vi "Open Connection (ODBC).vi"(8 "error in (no error)":errorcluster, 9 "password":string, 10 "userID":string, 11 "DSN Name":string) -> (0 "error out":errorcluster, 3 "connection reference":T1)   [LabVIEW 2020, in "Oracle Driver.lvlib"]
uses:
  Oracle Driver.lvlib
  <vilib>/addons/database/Connection.llb/Conn ObjectReference.ctl
  <vilib>/addons/database/Connection.llb/DB Tools Open Connec (String).vi
  <vilib>/addons/database/NI_Database_API.lvlib
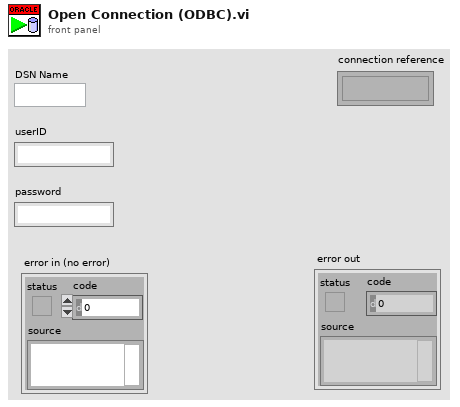
[diagram p1: front panel]
types:
  T1 = typedef "NI_Database_API.lvlib/Conn ObjectReference.ctl" = refnum<k1>
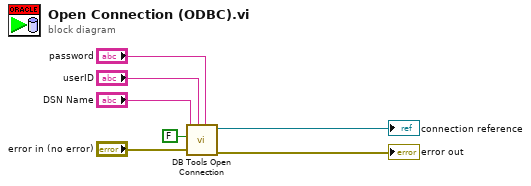
[diagram p0: block diagram]
diagram:
  n1 = call-poly <vilib>:"DB Tools Open Connection.vi"("password"="password", "userID"="userID", "error in (no error)"="error in (no error)", "prompt? (F)"=FALSE, "connection information"="DSN Name") -> ("error out"=→"error out":errorcluster, "connection reference"=→"connection reference":T1)  [unwired: 3 in]
